vi "Comprar.vi"(8 "error in (no error)":errorcluster, 10 "Productos 2":i32(listbox), 11 "Coca Actor in":refnum<class "Coca Actor.lvclass">) -> (0 "error out":errorcluster, 3 "Coca Actor out":refnum<class "Coca Actor.lvclass">)   [LabVIEW 2020, in "Coca Actor.lvlib" / "Coca Actor.lvclass"]
uses:
  Coca Actor.lvclass
  C:/Program Files (x86)/National Instruments/LabVIEW 2020/vi.lib/ActorFramework/Actor/Actor.lvclass
  <vilib>/ActorFramework/Actor/Actor.lvclass/Actor.ctl
  Coca Actor.lvclass/Coca Actor.ctl
  UI Actor Messages/Comparar precios Coca Msg/Comparar precios Coca Msg.lvclass/Comparar precios Coca Msg.ctl
  <vilib>/ActorFramework/Message Enqueuer/Message Enqueuer.lvclass/Message Enqueuer.ctl
  <vilib>/ActorFramework/Message Enqueuer/Enqueue.vi
  UI Actor Messages/Comparar precios Coca Msg/Comparar precios Coca Msg.lvclass
  C:/Program Files (x86)/National Instruments/LabVIEW 2020/vi.lib/ActorFramework/Message/Message.lvclass
  <vilib>/ActorFramework/Message Priority Queue/Priority Enqueue.vi
  <vilib>/ActorFramework/Actor/Actor.lvclass
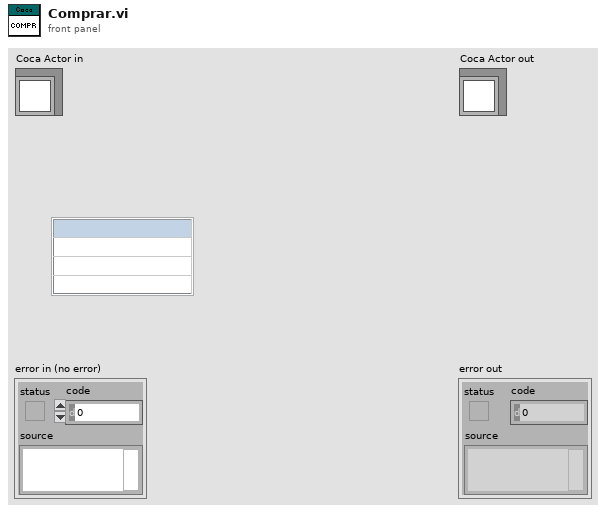
[diagram p1: front panel]
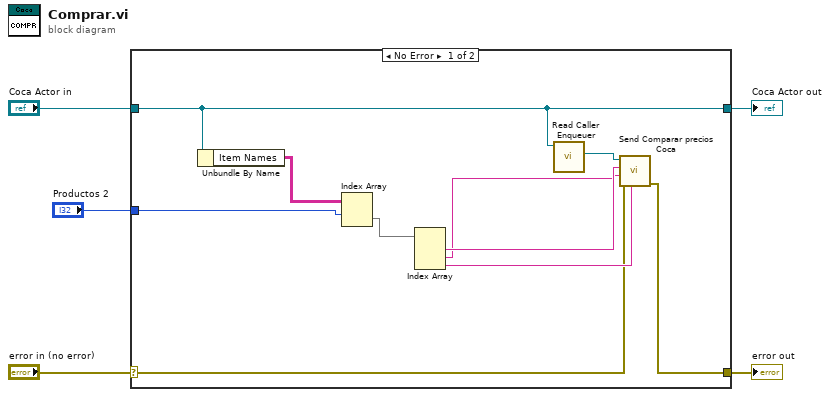
[diagram p0: block diagram]
diagram:
  n1 = case shown="No Error" "error in (no error)" {
    selector: "error in (no error)" -> [w7 w17]
    tunnel: [w6 w17] -> w4
    tunnel: [w12 w16] -> w2
    tunnel: "Coca Actor in" -> [w12 w16]
    tunnel: "Productos 2" -> [w14 _]
    frame No Error {
      n2 = Unbundle By Name(w12) -> ("Item Names"=w15:string[][])
      n3 = Index Array(array=w15, index (row)=w14) -> (element=w13:string[])  [unwired: 1 in]
      n4 = Index Array(array=w13) -> (element #1=w10:string, element #2=w9:string, element #3=w8:string)  [unwired: 3 in]
      n5 = call <vilib>:"Read Caller Enqueuer.vi"("Actor"=w12) -> ("Caller Enqueuer"=w11:refnum<class "Message Enqueuer.lvclass">)  [unwired: 10 in]
      n6 = call "Send Comparar precios Coca.vi"("Inventario"=w8, "error in (no error)"=w7, "Precio"=w9, "Producto"=w10, "Message Enqueuer"=w11) -> ("error out"=w6:errorcluster)  [unwired: 5 in, 1 out]
    }
    frame Error {
    }
  }
  "error out" <- w4
  "Coca Actor out" <- w2
